vi "界面2-数据采集.vi"() -> ()   [LabVIEW 2013]
uses:
  GlobleVar/SamplingRate.vi
  GlobleVar/segment_size.vi
panel:
  out "CH2输出电流":dbl format="%.1f mA"
  in  "输出增益百分比-显示":dbl format="%.1f %"
  out "CH1输出电流":dbl format="%.1f mA"
  in  "DEH类型发送":bool
  in  "DEH内置参数发送":bool
  in  "DEH内置参数值":dbl caption="内置参数值" format="%.1f %"
  in  "DEH类型":enum32{"内置", "外接"}(radio) caption="类型"
  in  "无输出":bool
  in  "阀门全关":bool
  in  "阀门全开":bool
  in  "输出增益百分比":sgl(slide) scale=0.0..100.0
  out "total_size":dbl format="%#_6p"
  in  "采集结束":bool
  out "Boolean":bool
  in  "试验结果->":bool
  in  "<-项目":bool
  in  "中止":bool
  in  "开始":bool
  in  "完成":bool
  out "采集进度":u8 format="%0.0f%%"
  out "采集\n进度":u8(slide) scale=0.0..100.0
  in  "采样时间":dbl=4.0 format="%#_g s"
  in  "试验模式":u16(ring) items=["快关L1L2", "快关L1", "快关L2", "步响应1", "归零", "开启关闭"]
  out "实时采集":cluster{dbl, dbl, dbl[][]}(graph)
  # "DEH"
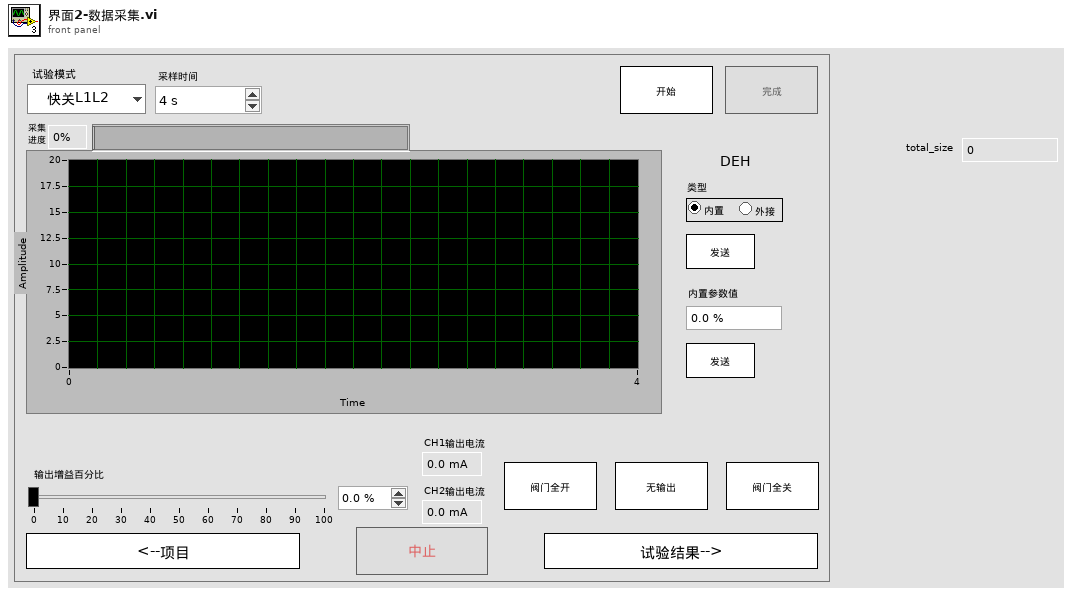
[diagram p1: front panel]
types:
  T1 = enum16{"初始化", "等待事件", "退出", "数据采集", "数据处理", "开启阀门"}
  T2 = cluster{"联机状态":bool, "外置清零信号":bool, "卡件工作模式":enum16{"无输出", "正常工作", "阀门常开", "阀门常闭"}, "卡件序列号":string, "卡件物理地址":string, "伺服阀输出电流CH1":dbl, "输出通道状态CH1":bool, "伺服阀输出电流CH2":dbl, "输出通道状态CH2":bool, "伺服输出使能CH1 ":bool, "伺服输出使能CH2":bool, "LVDT1类型":enum16{"未接入", "直流", "交流"}, "LVDT1直流回路":bool, "LVDT1次级线圈 2":bool, "LVDT1次级线圈 1":bool, "LVDT1初级线圈":bool, "LVDT2类型":enum16{"未接入", "直流", "交流"}, "LVDT2直流回路":bool, "LVDT2次级线圈 2":bool, "LVDT2次级线圈 1":bool, "LVDT2初级线圈":bool, "DEH回路状态":bool, "DEH类型":enum16{"内置", "外接"}, "转速反馈使能":bool, "LVDT1信号采样百分比":dbl, "LVDT2信号采样百分比":dbl, "DEH指令值":u8, "转速差反馈量":dbl, "回路1转速":dbl, "回路2转速":dbl, "回路3转速":dbl, "中选转速":dbl, "LVDT1 ADC":i16, "LVDT2 ADC":i16, "DEH ADC":i16, "LVDT1ZADC":i16, "LVDT2ZADC":i16, "LVDT1FADC":i16, "LVDT2FADC":i16, "DehZeroCali":bool, "DehFullCali":bool, "LVDT1ZeroCali":bool, "LVDT1FullCali":bool, "LVDT2ZeroCali":bool, "LVDT2FullCali":bool, "转速零度标定":i16, "转速满度标定":i16, "转速指令采样值":i16, "标准转速":dbl}
  T3 = enum8{"Enabled", "Disabled", "Disabled and Grayed Out"}
  T4 = enum16{"open", "open or create", "create or replace", "create", "open (read-only)"}
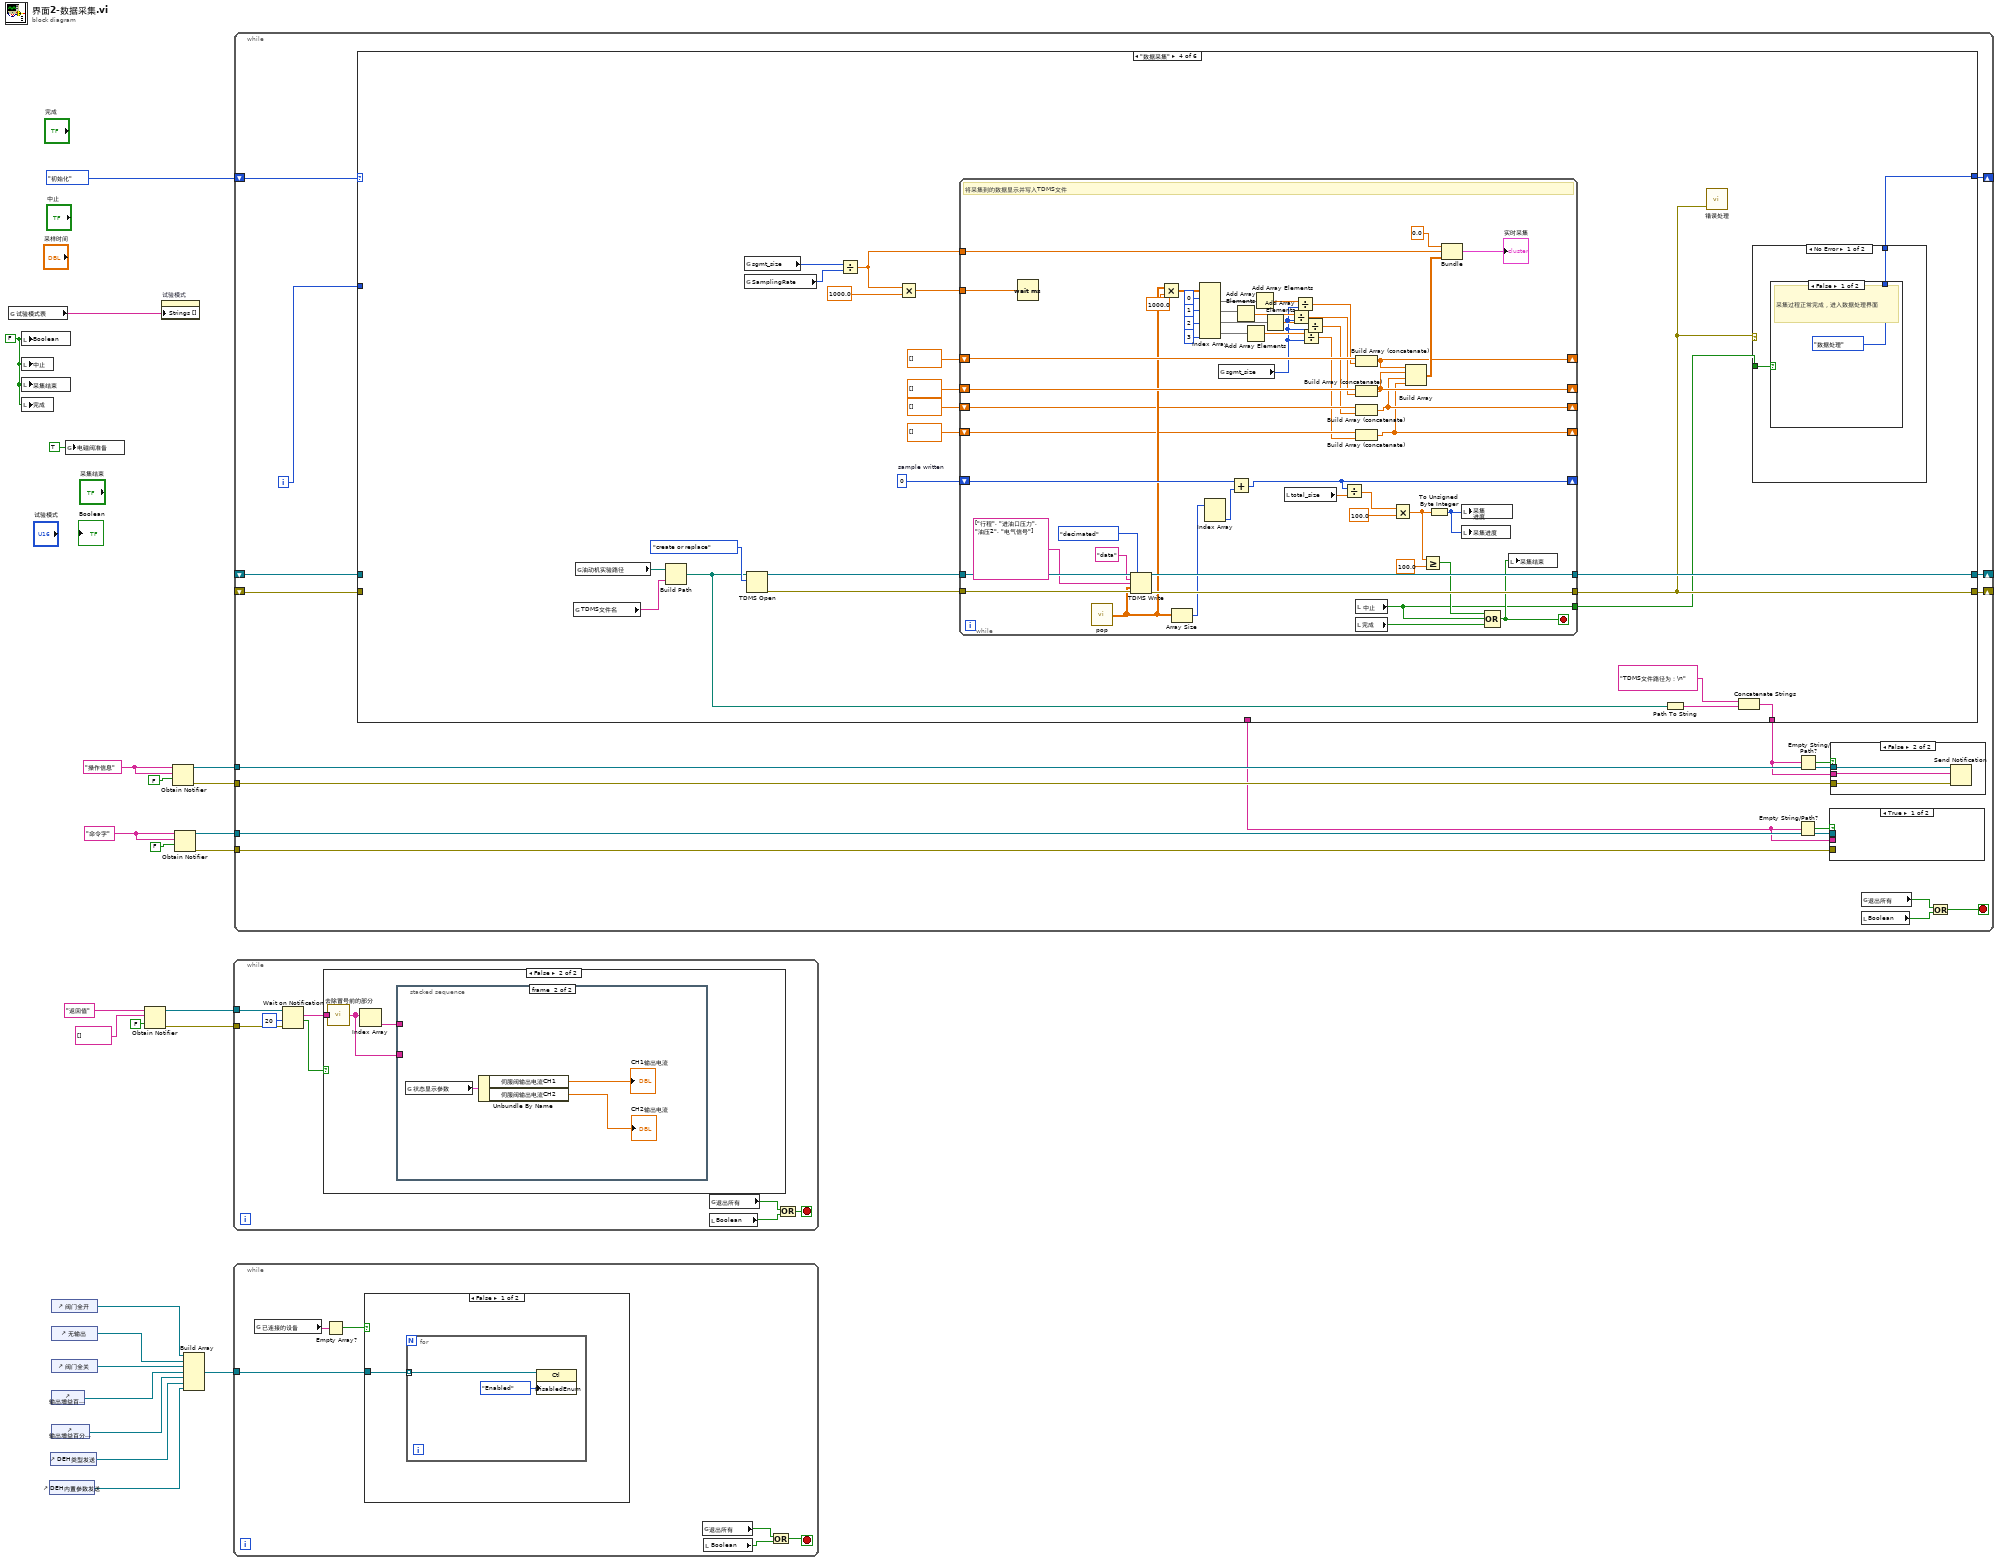
[diagram p0: block diagram]
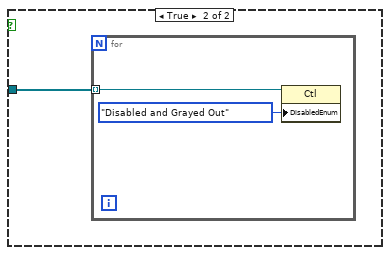
[diagram p2: hidden frame]
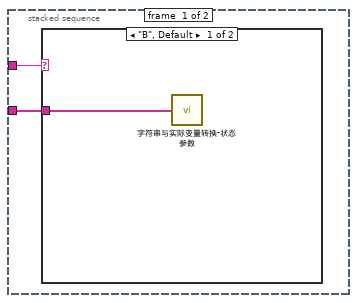
[diagram p4: hidden frame]
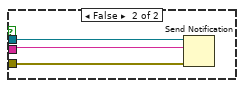
[diagram p6: hidden frame]
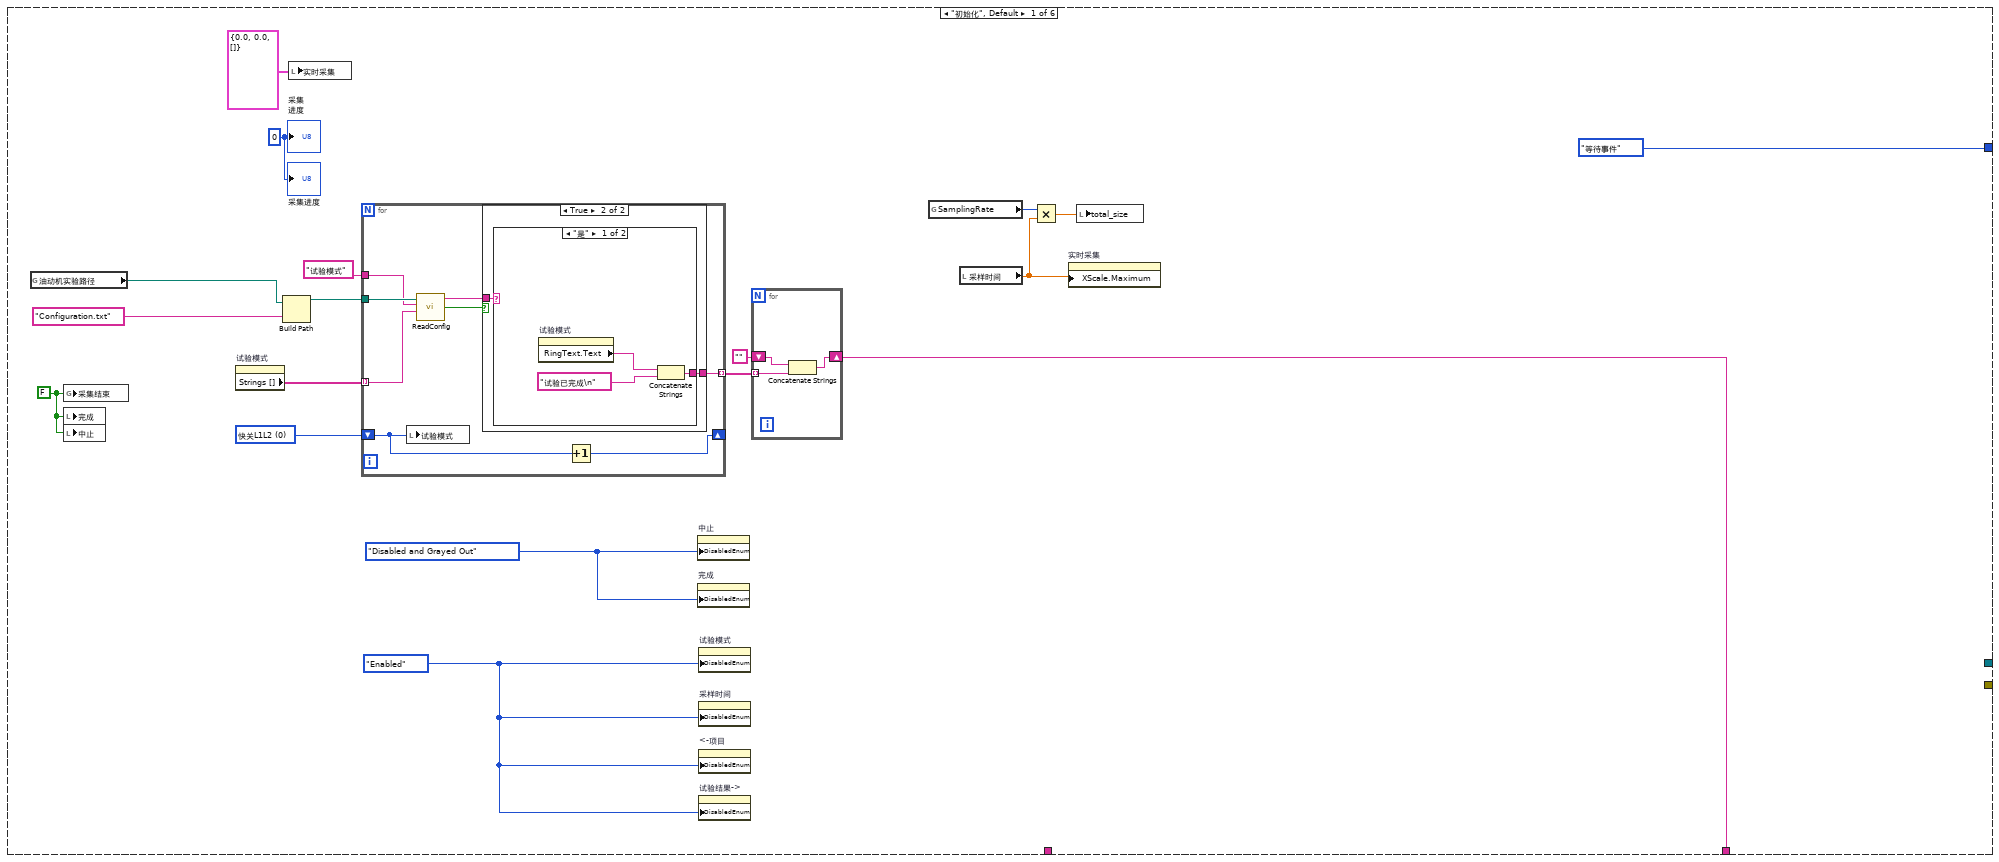
[diagram p8: hidden frame]
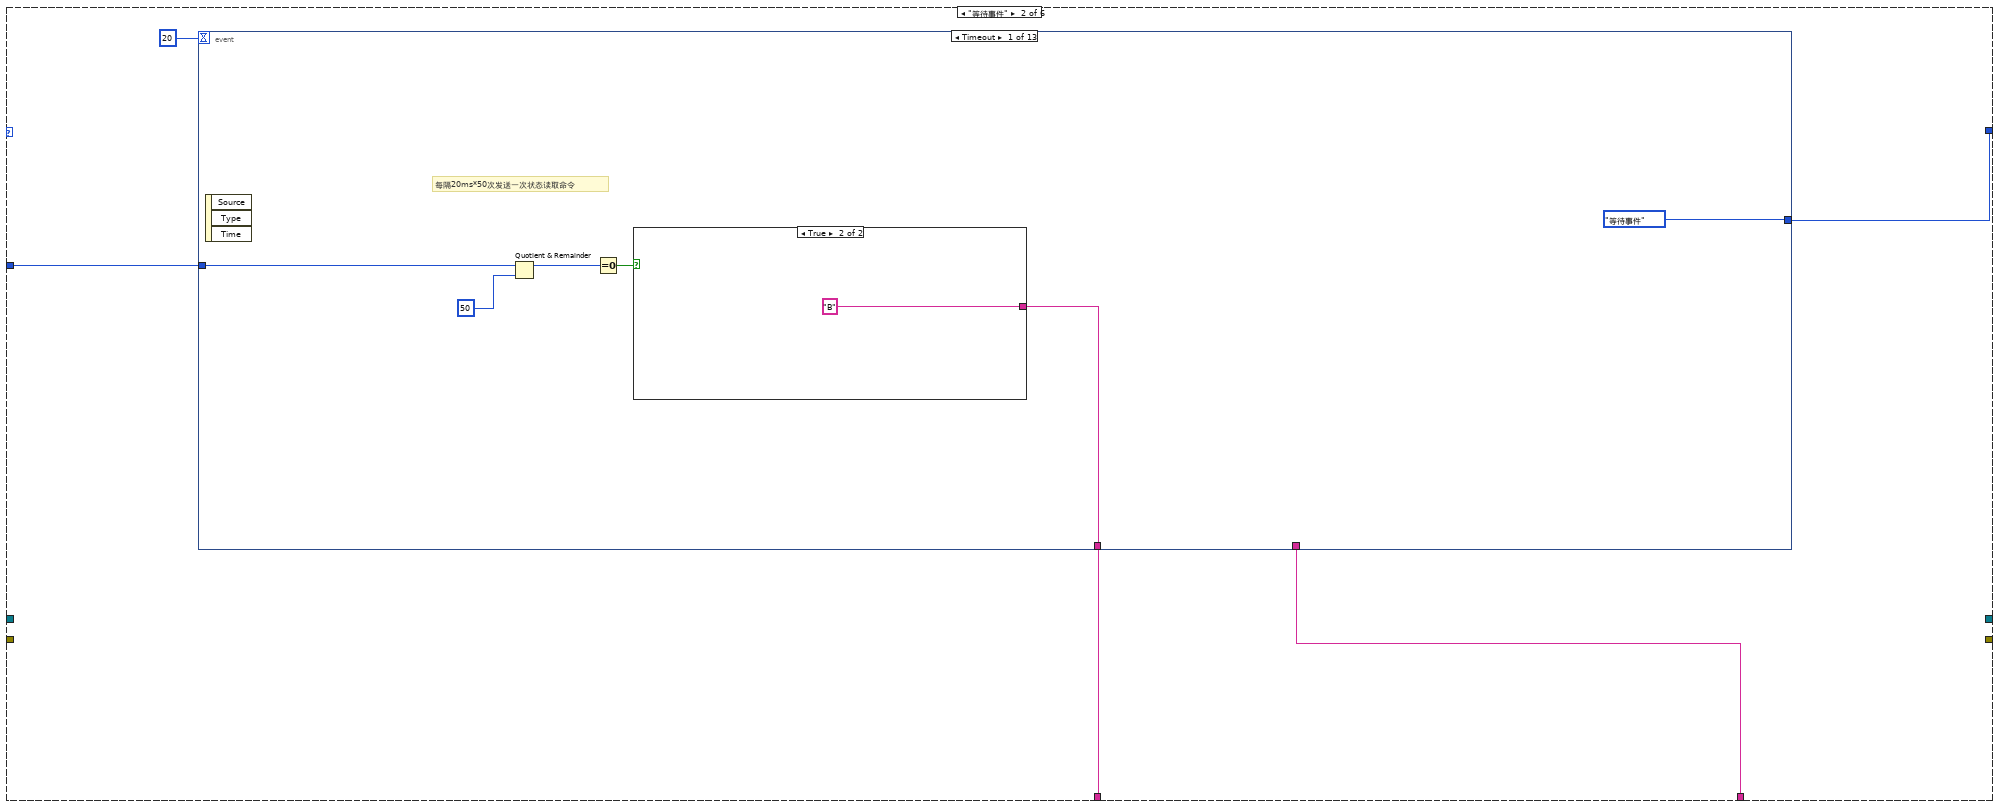
[diagram p11: hidden frame]
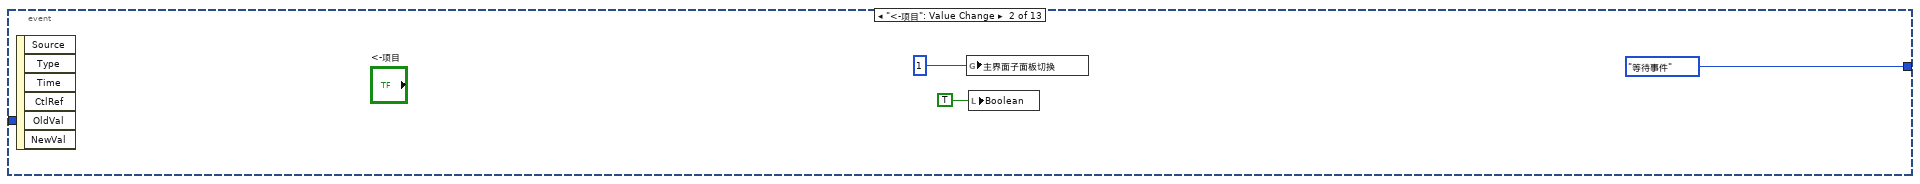
[diagram p13: hidden frame]
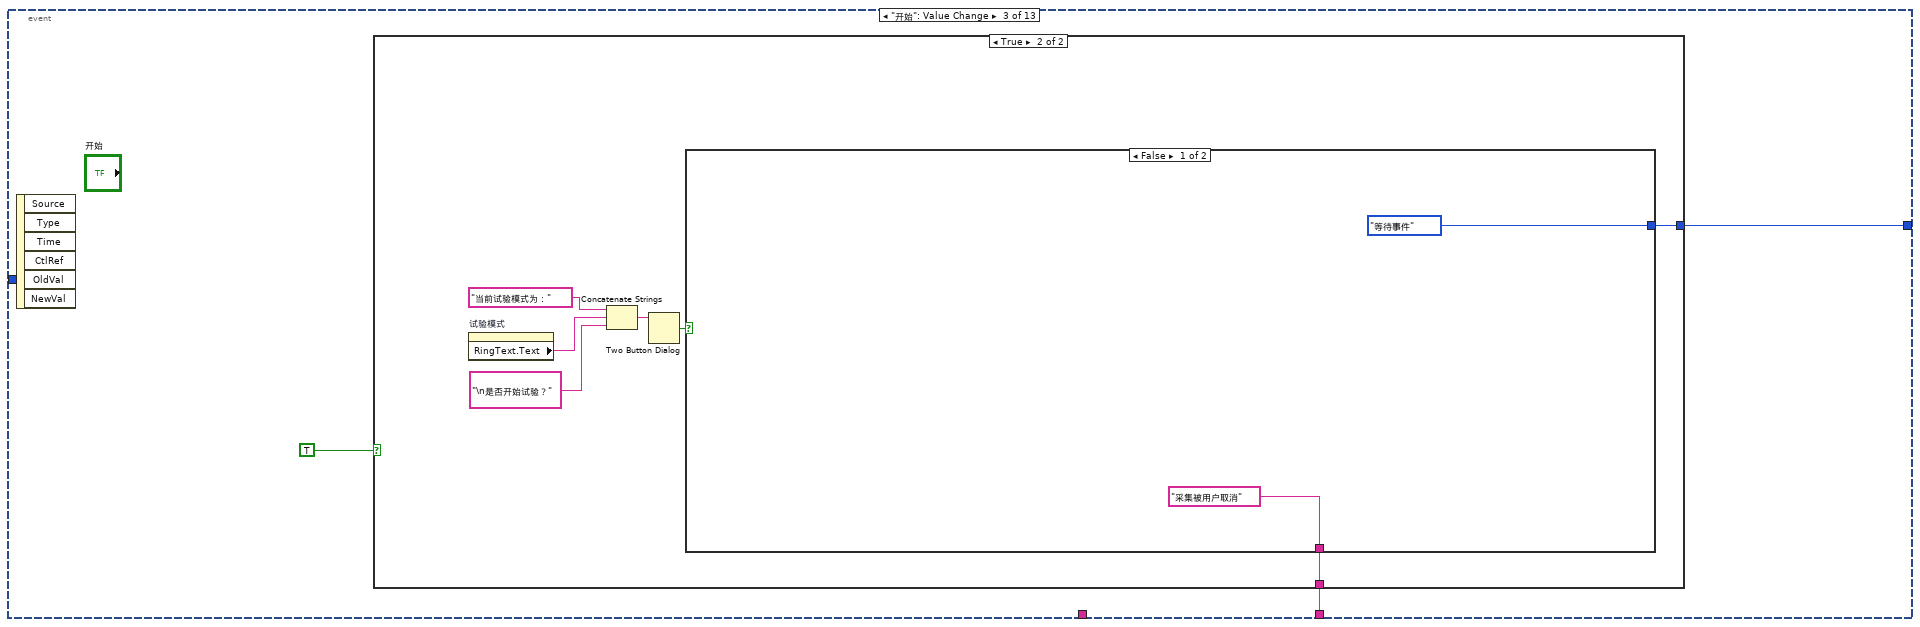
[diagram p14: hidden frame]
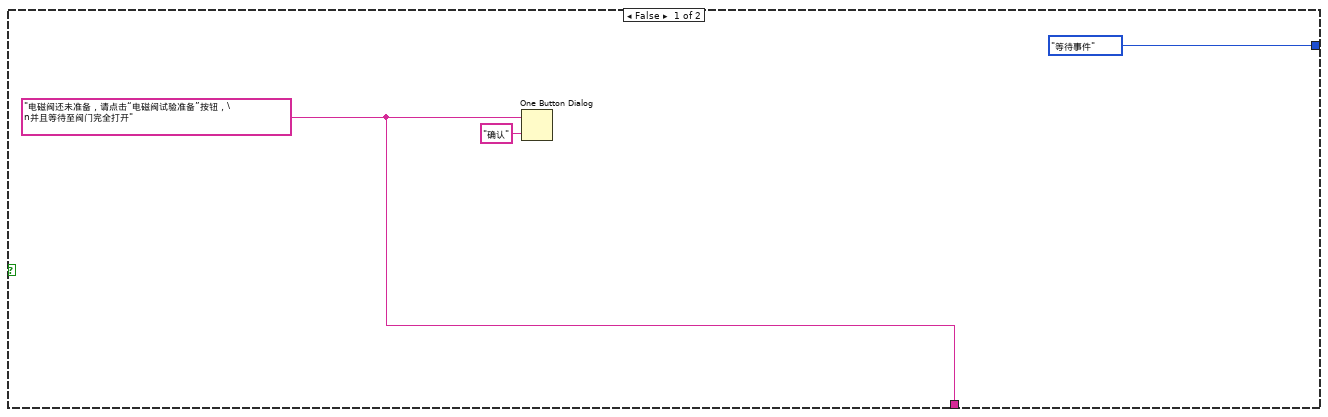
[diagram p15: hidden frame]
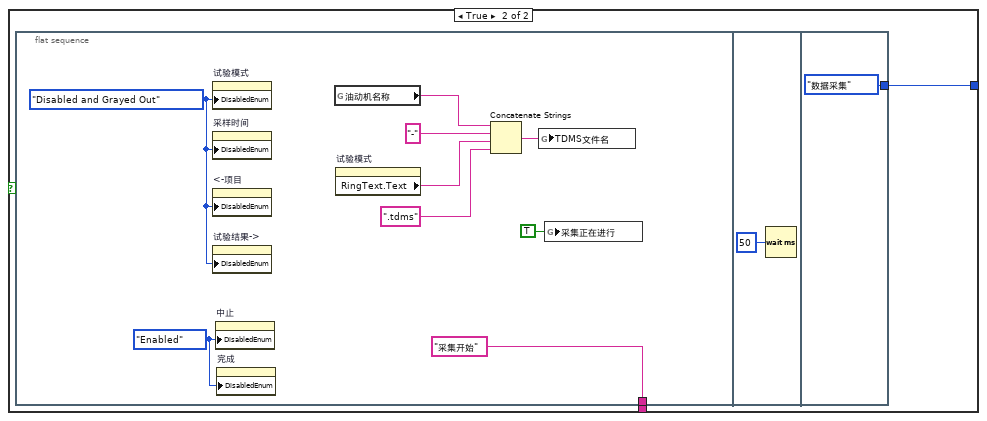
[diagram p16: hidden frame]
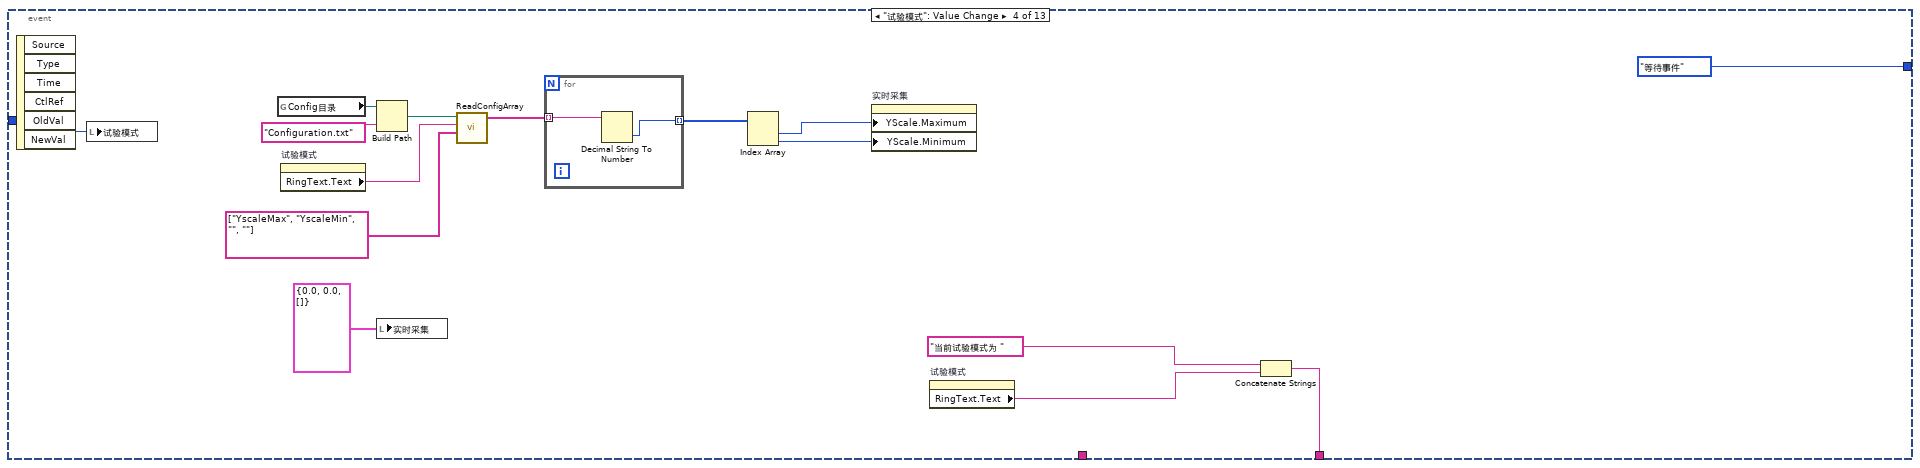
[diagram p17: hidden frame]
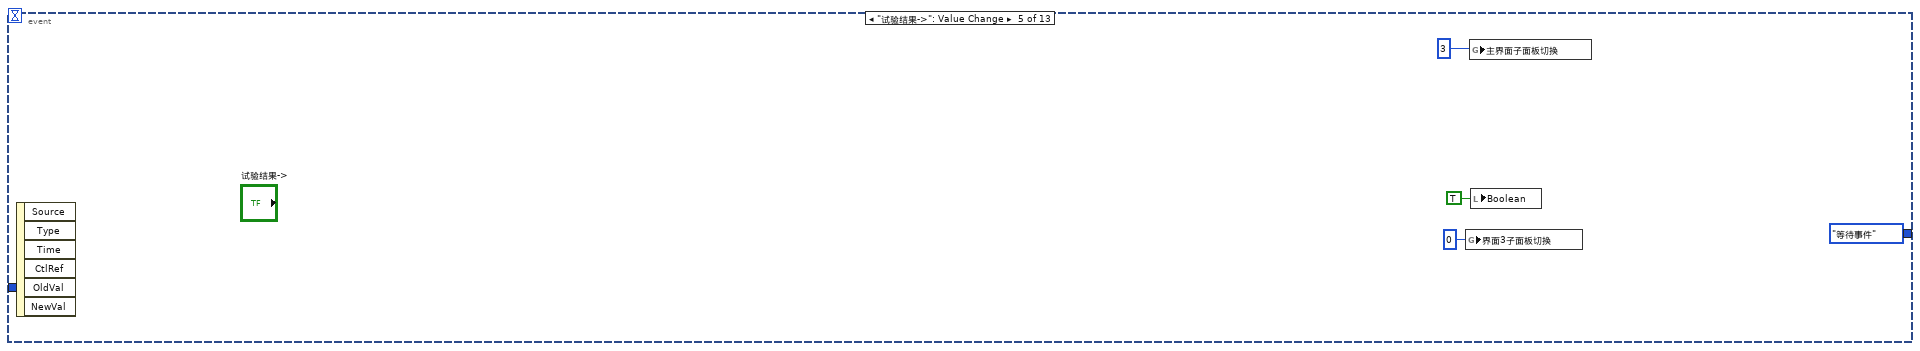
[diagram p18: hidden frame]
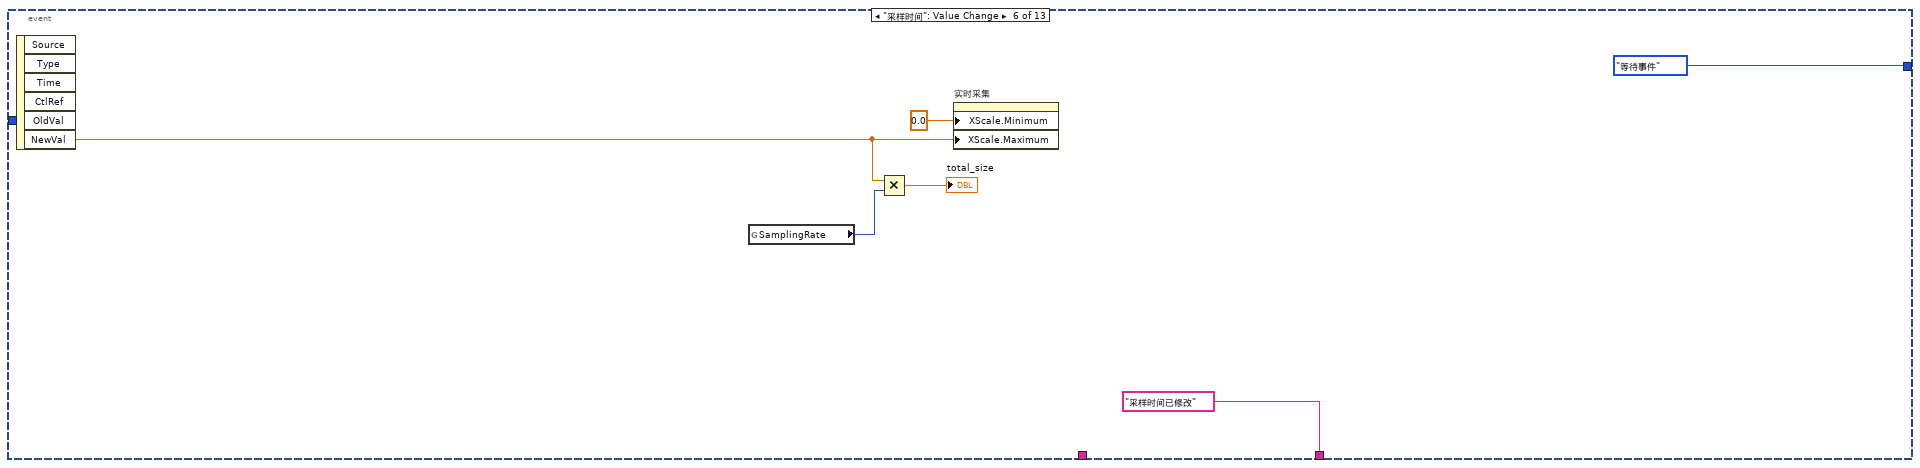
[diagram p19: hidden frame]
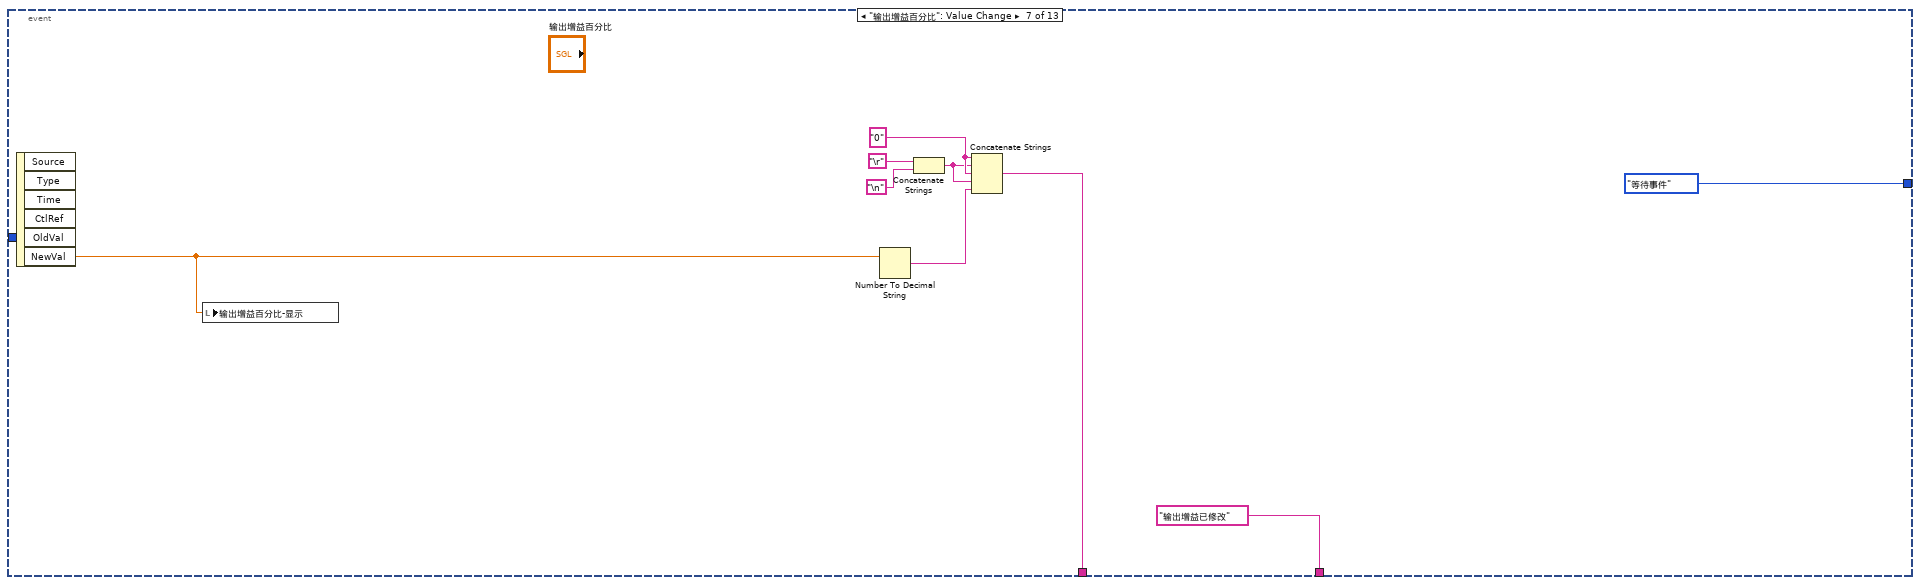
[diagram p20: hidden frame]
diagram:
  w16 = "命令字"
  w19 = FALSE ("Boolean")
  w24 = "操作信息"
  n1 = global read "试验模式表.vi" "试验模式表"() -> (w20:string[])
  n2 = local write "Boolean"(w19) -> ()
  n3 = local write "中止"(w19) -> ()
  n4 = local write "采集结束"(w19) -> ()
  n5 = local write "完成"(w19) -> ()
  n6 = control-ref of="DEH内置参数发送"() -> (w1:refnum<vi>)
  n7 = control-ref of="DEH类型发送"() -> (w2:refnum<vi>)
  n8 = control-ref of="阀门全开"() -> (w8:refnum<vi>)
  n9 = control-ref of="无输出"() -> (w7:refnum<vi>)
  n10 = control-ref of="阀门全关"() -> (w6:refnum<vi>)
  n11 = control-ref of="输出增益百分比"() -> (w5:refnum<vi>)
  n12 = control-ref of="输出增益百分比-显示"() -> (w4:refnum<vi>)
  n13 = global write "电磁阀准备.vi" "电磁阀准备"(TRUE ("电磁阀准备")) -> ()
  n14 = Obtain Notifier(name (unnamed)="返回值", notification data type=string[] [], create if not found? (T)=FALSE) -> (notifier out=w11:refnum<notifier>, error out=w10:errorcluster)  [unwired: 1 in, 1 out]
  n15 = property on="试验模式" class="Ring (strict)"("Strings []"=w20) -> ()  [unwired: 2 in, 2 out]
  n16 = Obtain Notifier(name (unnamed)=w24, notification data type=w24, create if not found? (T)=FALSE) -> (notifier out=w23:refnum<notifier>, error out=w22:errorcluster)  [unwired: 1 in, 1 out]
  n17 = Obtain Notifier(name (unnamed)=w16, notification data type=w16, create if not found? (T)=FALSE) -> (notifier out=w15:refnum<notifier>, error out=w14:errorcluster)  [unwired: 1 in, 1 out]
  n18 = Build Array(w8, w7, w6, w5, w4, w2, w1) -> (w3:refnum<vi>[])
  n19 = while {
    tunnel: w11 -> [w32]
    tunnel: w10 -> [w31]
    stop <- w28 stop-if-true
    n20 = Wait on Notification(notifier=w32, timeout in ms (-1)=20, error in (no error)=w31) -> (notification=w30:string[], timed out?=w26:bool)  [unwired: 1 in, 2 out]
    n21 = case shown="False" w26 {
      tunnel: w30 -> [_ w36]
      frame True {
      }
      frame False {
        n22 = call "去除冒号前的部分.vi"("返回值列表"=w36) -> ("返回值参数列表"=w34:string[])
        n23 = Index Array(array=w34) -> (element=w35:string)  [unwired: 1 in]
        n24 = stacked-sequence {
          tunnel: w35 -> [w38 _]
          tunnel: w34 -> [w37 _]
          frame #0 {
            n25 = case shown="\"B\", Default" w38 {
              tunnel: w37 -> [w39 _]
              frame "B", Default {
                n26 = call "字符串与实际变量转换-状态参数.vi"("状态参数"=w39) -> ()  [unwired: 5 in]
              }
              frame "True" {
              }
            }
          }
          frame #1 {
            n27 = global read "状态显示参数.vi" "状态显示参数"() -> (w42:T2)
            n28 = Unbundle By Name(w42) -> ("伺服阀输出电流CH1"=→"CH1输出电流":dbl, "伺服阀输出电流CH2"=→"CH2输出电流":dbl)
          }
        }
      }
    }
    n29 = global read "退出所有.vi" "退出所有"() -> (w29:bool)
    n30 = local read "Boolean"() -> (w27:bool)
    n31 = Or(x=w29, y=w27) -> (x .or. y?=w28:bool)
  }
  n32 = while {
    tunnel: w3 -> [w46]
    stop <- w44 stop-if-true
    n33 = global read "已连接的设备.vi" "已连接的设备"() -> (w48:string[])
    n34 = Empty Array?(array=w48) -> (empty?=w47:bool)
    n35 = case shown="False" w47 {
      tunnel: w46 -> [w49 w52]
      frame False {
        n36 = for {
          tunnel: w49 -> [w51] mode=indexing
          n37 = property class="Ctl"(reference=w51, "DisabledEnum"=T3."Enabled" ("Disabled")) -> ()  [unwired: 1 in, 2 out]
        }
      }
      frame True {
        n38 = for {
          tunnel: w52 -> [w54] mode=indexing
          n39 = property class="Ctl"(reference=w54, "DisabledEnum"=T3."Disabled and Grayed Out" ("Disabled")) -> ()  [unwired: 1 in, 2 out]
        }
      }
    }
    n40 = global read "退出所有.vi" "退出所有"() -> (w45:bool)
    n41 = local read "Boolean"() -> (w43:bool)
    n42 = Or(x=w45, y=w43) -> (x .or. y?=w44:bool)
  }
  n43 = while {
    shift-right: [w70] -> _
    shift-left: T1."初始化" -> [w71]
    tunnel: w23 -> [w72]
    tunnel: w22 -> [w60]
    shift-right: [w64] -> _
    shift-left: _ -> [w62]
    shift-right: [w63] -> _
    shift-left: _ -> [w61]
    tunnel: w15 -> [w58]
    tunnel: w14 -> [w56]
    i -> [w55]
    stop <- w67 stop-if-true
    n44 = case shown="\"数据采集\"" w71 {
      tunnel: [w86 w116 w253 w281 "数据处理完成" "阀门已开启"] -> w65
      tunnel: [enum16{"初始化", "等待事件", "退出"}."等待事件" w117 T1."初始化" w282 T1."等待事件" T1."数据采集"] -> w70
      tunnel: [_ _ _ w283 _ _] -> w64
      tunnel: [_ _ _ w280 _ _] -> w63
      tunnel: w62 -> [_ _ w255 _ w353 _]
      tunnel: w61 -> [_ _ w254 _ w352 _]
      tunnel: [_ w114 _ _ _ _] -> w57
      tunnel: w55 -> [_ w113 _ _ _ _]
      frame "初始化", Default {
        w82 = T3."Disabled and Grayed Out" ("Disabled")
        w83 = T3."Enabled" ("Disabled")
        w89 = u16 0 items=["快关L1L2", "快关L1", "快关L2", "步响应", "归零", "开启关闭", ""] ("试验模式")
        w85 = FALSE
        w95 = u8 0 ("采集\n进度")
        n45 = global read "油动机实验路径.vi" "油动机实验路径"() -> (w93:path)
        n46 = global write "采集结束.vi" "采集结束"(w85) -> ()
        n47 = local write "完成"(w85) -> ()
        n48 = local write "中止"(w85) -> ()
        n49 = property on="试验模式" class="Ring (strict)"() -> ("Strings []"=w90:string[])  [unwired: 2 in, 2 out]
        n50 = Build Path(base path=w93, name or relative path="Configuration.txt" ("名称或相对路径")) -> (appended path=w92:path)
        n51 = local write "实时采集"(cluster{dbl, dbl, dbl[][]} {0.0, 0.0, []} ("实时采集")) -> ()
        n52 = for {
          tunnel: w92 -> [w107]
          tunnel: "试验模式" -> [w106]
          tunnel: w90 -> [w105] mode=indexing
          shift-right: [w101] -> _
          shift-left: w89 -> [w102]
          tunnel: [w100] -> w87 mode=indexing
          n53 = local write "试验模式"(w102) -> ()
          n54 = call "ReadConfig.vi"("Key"=w105, "Section"=w106, "Path"=w107) -> ("Key found?"=w104:bool, "Value"=w103:string)  [unwired: 1 in, 1 out]
          n55 = case shown="True" w104 {
            tunnel: w103 -> [_ w109]
            tunnel: [_ w108] -> w100
            frame False {
            }
            frame True {
              n56 = case shown="\"是\"" w109 {
                tunnel: [w110 _] -> w108
                frame "是" {
                  n57 = property on="试验模式" class="Ring (strict)"() -> ("RingText.Text"=w111:string)  [unwired: 2 in, 2 out]
                  n58 = Concatenate Strings(w111, "试验已完成\n") -> (w110:string)
                }
                frame "否", Default {
                }
              }
            }
          }
          n59 = Increment(x=w102) -> (x+1=w101:u16)
        }
        n60 = property on="中止" class="Bool (strict)"("DisabledEnum"=w82) -> ()  [unwired: 2 in, 2 out]
        n61 = property on="完成" class="Bool (strict)"("DisabledEnum"=w82) -> ()  [unwired: 2 in, 2 out]
        n62 = property on="试验模式" class="Ring (strict)"("DisabledEnum"=w83) -> ()  [unwired: 2 in, 2 out]
        n63 = property on="采样时间" class="DigNum (strict)"("DisabledEnum"=w83) -> ()  [unwired: 2 in, 2 out]
        n64 = property on="<-项目" class="Bool"("DisabledEnum"=w83) -> ()  [unwired: 2 in, 2 out]
        n65 = property on="试验结果->" class="Bool"("DisabledEnum"=w83) -> ()  [unwired: 2 in, 2 out]
        n66 = for {
          shift-right: [w97] -> w86
          shift-left: "" -> [w98]
          tunnel: w87 -> [w99] mode=indexing
          n67 = Concatenate Strings(w98, w99) -> (w97:string)
        }
        n68 = global read "SamplingRate.vi" "SamplingRate"() -> (w79:i32)
        n69 = local read "采样时间"() -> (w80:dbl)
        n70 = Multiply(x=w79, y=w80) -> (x*y=w81:dbl)
        n71 = property on="实时采集" class="WFGraph (strict)"("XScale.Maximum"=w80) -> ()  [unwired: 2 in, 2 out]
        n72 = local write "total_size"(w81) -> ()
        "采集\n进度" <- w95
        "采集进度" <- w95
      }
      frame "等待事件" {
        n73 = event shown="[0] Timeout" {
          selector: _ -> [_ _ _ _ _ _ _ _ _ _ _ _ _]
          dyn-events: _ -> [_ _ _ _ _ _ _ _ _ _ _ _ _]
          timeout: 20 -> [_ _ _ _ _ _ _ _ _ _ _ _ _]
          tunnel: [T1."等待事件" T1."等待事件" w130 T1."等待事件" T1."等待事件" T1."等待事件" T1."等待事件" T1."等待事件" T1."等待事件" T1."等待事件" T1."等待事件" T1."等待事件" T1."等待事件"] -> w117
          tunnel: [_ _ w129 w167 _ "采样时间已修改" "输出增益已修改" ("消息") "输出增益已修改" ("消息") "无输出命令已发送" ("消息") "阀门全开命令已发送" ("消息") "阀门全关命令已发送" ("消息") w229 "DEH内置参数已发送" ("消息")] -> w116
          tunnel: [w118 _ _ _ _ _ w186 w195 w203 w218 w221 w234 w246] -> w114
          tunnel: w113 -> [w122 _ _ _ _ _ _ _ _ _ _ _ _]
          event Timeout {
            # "每隔20ms*50次发送一次状态读取命令"
            n74 = event-data() -> ()  [unwired: 1 in, 3 out]
            n75 = Quotient & Remainder(x=w122, y=50) -> (x-y*floor(x/y)=w119:i32)  [unwired: 1 out]
            n76 = Equal To 0?(x=w119) -> (x = 0?=w120:bool)
            n77 = case shown="True" w120 {
              tunnel: [_ "B"] -> w118
              frame False {
              }
              frame True {
              }
            }
          }
          event "<-项目": Value Change {
            n78 = event-data() -> ()  [unwired: 1 in, 6 out]
            n79 = global write "主界面子面板切换.vi" "主界面子面板切换"(1) -> ()
            n80 = local write "Boolean"(TRUE ("Boolean")) -> ()
          }
          event "开始": Value Change {
            n81 = event-data() -> ()  [unwired: 1 in, 6 out]
            n82 = case shown="True" TRUE {
              tunnel: [T1."等待事件" w140] -> w130
              tunnel: [w131 w134] -> w129
              frame False {
                w131 = "电磁阀还未准备，请点击“电磁阀试验准备”按钮，\n并且等待至阀门完全打开" ("消息")
                n83 = One Button Dialog(message=w131, button name ("OK")="确认") -> ()  [unwired: 1 out]
              }
              frame True {
                n84 = property on="试验模式" class="Ring (strict)"() -> ("RingText.Text"=w138:string)  [unwired: 2 in, 2 out]
                n85 = Concatenate Strings("当前试验模式为：", w138, "\n是否开始试验？") -> (w136:string)
                n86 = Two Button Dialog(message=w136) -> (T button?=w135:bool)  [unwired: 2 in]
                n87 = case shown="False" w135 {
                  tunnel: [T1."等待事件" w143] -> w140
                  tunnel: ["采集被用户取消" w144] -> w134
                  frame False {
                  }
                  frame True {
                    n88 = flat-sequence {
                      tunnel: ["采集开始"] -> w144
                      tunnel: [T1."数据采集"] -> w143
                      frame #0 {
                        w146 = T3."Enabled" ("Disabled")
                        w147 = T3."Disabled and Grayed Out" ("Disabled")
                        n89 = property on="试验模式" class="Ring (strict)"("DisabledEnum"=w147) -> ()  [unwired: 2 in, 2 out]
                        n90 = property on="采样时间" class="DigNum (strict)"("DisabledEnum"=w147) -> ()  [unwired: 2 in, 2 out]
                        n91 = property on="<-项目" class="Bool"("DisabledEnum"=w147) -> ()  [unwired: 2 in, 2 out]
                        n92 = property on="试验结果->" class="Bool"("DisabledEnum"=w147) -> ()  [unwired: 2 in, 2 out]
                        n93 = property on="中止" class="Bool (strict)"("DisabledEnum"=w146) -> ()  [unwired: 2 in, 2 out]
                        n94 = property on="完成" class="Bool (strict)"("DisabledEnum"=w146) -> ()  [unwired: 2 in, 2 out]
                        n95 = global read "油动机名称.vi" "油动机名称"() -> (w149:string)
                        n96 = property on="试验模式" class="Ring (strict)"() -> ("RingText.Text"=w151:string)  [unwired: 2 in, 2 out]
                        n97 = Concatenate Strings(w149, "-", w151, ".tdms") -> (w153:string)
                        n98 = global write "TDMS文件名.vi" "TDMS文件名"(w153) -> ()
                        n99 = global write "采集正在进行.vi" "采集正在进行"(TRUE ("采集正在进行")) -> ()
                      }
                      frame #1 {
                        n100 = Wait (ms)(milliseconds to wait=u32 50) -> ()  [unwired: 1 out]
                      }
                      frame #2 {
                      }
                    }
                  }
                }
              }
            }
          }
          event "试验模式": Value Change {
            n101 = event-data() -> ("NewVal"=w170:u16)  [unwired: 1 in, 5 out]
            n102 = local write "试验模式"(w170) -> ()
            n103 = global read "Config目录.vi" "Config目录"() -> (w164:path)
            n104 = property on="试验模式" class="Ring (strict)"() -> ("RingText.Text"=w162:string)  [unwired: 2 in, 2 out]
            n105 = Build Path(base path=w164, name or relative path="Configuration.txt") -> (appended path=w165:path)
            n106 = local write "实时采集"(cluster{dbl, dbl, dbl[][]} {0.0, 0.0, []} ("实时采集")) -> ()
            n107 = call "ReadConfigArray.vi"("KeyArray"=string[] ["YscaleMax", "YscaleMin", "", ""], "Section"=w162, "Path"=w165) -> ("ValueArray"=w160:string[])  [unwired: 1 in, 2 out]
            n108 = for {
              tunnel: w160 -> [w172] mode=indexing
              tunnel: [w171] -> w159 mode=indexing
              n109 = Decimal String To Number(string=w172) -> (number=w171:i32)  [unwired: 2 in, 1 out]
            }
            n110 = Index Array(array=w159) -> (element #1=w158:i32, element #2=w157:i32)  [unwired: 2 in]
            n111 = property on="实时采集" class="WFGraph (strict)"("YScale.Maximum"=w158, "YScale.Minimum"=w157) -> ()  [unwired: 2 in, 2 out]
            n112 = property on="试验模式" class="Ring (strict)"() -> ("RingText.Text"=w168:string)  [unwired: 2 in, 2 out]
            n113 = Concatenate Strings("当前试验模式为 ", w168) -> (w167:string)
          }
          event "试验结果->": Value Change {
            n114 = event-data() -> ()  [unwired: 1 in, 6 out]
            n115 = global write "界面3子面板切换.vi" "界面3子面板切换"(0 ("界面3子面板切换")) -> ()
            n116 = global write "主界面子面板切换.vi" "主界面子面板切换"(3) -> ()
            n117 = local write "Boolean"(TRUE ("Boolean")) -> ()
          }
          event "采样时间": Value Change {
            n118 = event-data() -> ("NewVal"=w181:dbl)  [unwired: 1 in, 5 out]
            n119 = global read "SamplingRate.vi" "SamplingRate"() -> (w178:i32)
            n120 = Multiply(x=w181, y=w178) -> (x*y=→"total_size":dbl)
            n121 = property on="实时采集" class="WFGraph (strict)"("XScale.Minimum"=0.0 ("X Scale.Range:Minimum"), "XScale.Maximum"=w181) -> ()  [unwired: 2 in, 2 out]
          }
          event "输出增益百分比": Value Change {
            w189 = "0"
            n122 = event-data() -> ("NewVal"=w183:sgl)  [unwired: 1 in, 5 out]
            n123 = local write "输出增益百分比-显示"(w183) -> ()
            n124 = Number To Decimal String(number=w183) -> (decimal integer string=w187:string)  [unwired: 1 in]
            n125 = Concatenate Strings("\r", "\n") -> (w188:string)
            n126 = Concatenate Strings(w189, w188, w189, w188, w187) -> (w186:string)
          }
          event "输出增益百分比-显示": Value Change {
            w198 = "0"
            n127 = event-data() -> ("NewVal"=w194:dbl)  [unwired: 1 in, 5 out]
            n128 = local write "输出增益百分比"(w194) -> ()
            n129 = Number To Decimal String(number=w194) -> (decimal integer string=w196:string)  [unwired: 1 in]
            n130 = Concatenate Strings("\r", "\n") -> (w197:string)
            n131 = Concatenate Strings(w198, w197, w198, w197, w196) -> (w195:string)
          }
          event "无输出": Value Change {
            n132 = event-data() -> ()  [unwired: 1 in, 6 out]
            n133 = Concatenate Strings("\r", "\n") -> (w206:string)
            n134 = Concatenate Strings("0", w206, "1", w206, "0") -> (w203:string)
          }
          event "阀门全开": Value Change {
            n135 = event-data() -> ()  [unwired: 1 in, 6 out]
            n136 = Concatenate Strings("\r", "\n") -> (w214:string)
            n137 = Concatenate Strings("0", w214, "1", w214, "2") -> (w218:string)
          }
          event "阀门全关": Value Change {
            n138 = event-data() -> ()  [unwired: 1 in, 6 out]
            n139 = Concatenate Strings("\r", "\n") -> (w224:string)
            n140 = Concatenate Strings("0", w224, "1", w224, "3") -> (w221:string)
          }
          event "DEH类型发送": Value Change {
            n141 = event-data() -> ()  [unwired: 1 in, 6 out]
            n142 = Number To Decimal String(number="DEH类型") -> (decimal integer string=w233:string)  [unwired: 1 in]
            n143 = Concatenate Strings("\r", "\n") -> (w236:string)
            n144 = Concatenate Strings("0", w236, "2", w236, w233) -> (w234:string)
            n145 = case shown="\"外接\"" "DEH类型" {
              tunnel: ["内置" "外接"] -> w230
              frame "内置", Default {
              }
              frame "外接" {
              }
            }
            n146 = Concatenate Strings("DEH设置为：" ("消息"), w230) -> (w229:string)
          }
          event "DEH内置参数发送": Value Change {
            n147 = event-data() -> ()  [unwired: 1 in, 6 out]
            n148 = Number To Fractional String(number="DEH内置参数值") -> (F-format string=w244:string)  [unwired: 3 in]
            n149 = Concatenate Strings("\r", "\n") -> (w247:string)
            n150 = Concatenate Strings("5", w247, w244) -> (w246:string)
          }
        }
      }
      frame "退出" {
        w251 = T3."Disabled and Grayed Out" ("Disabled")
        w252 = T3."Enabled" ("Disabled")
        n151 = flat-sequence {
          tunnel: w255 -> [w259]
          tunnel: w254 -> [w258]
          tunnel: ["TDMS和TDMS_index已删除"] -> w253
          frame #0 {
            n152 = TDMS Close(8:w258, 11:w259) -> ()  [unwired: 2 out]
            n153 = Wait (ms)(milliseconds to wait=u32 20) -> ()  [unwired: 1 out]
          }
          frame #1 {
            n154 = global read "油动机实验路径.vi" "油动机实验路径"() -> (w261:path)
            n155 = global read "TDMS文件名.vi" "TDMS文件名"() -> (w268:string)
            n156 = Build Path(base path=w261, name or relative path=w268) -> (appended path=w263:path)
            n157 = Path To String(path=w263) -> (string=w262:string)
            n158 = Concatenate Strings(w262, "_index" ("字符串")) -> (w266:string)
            n159 = String To Path(string=w262) -> (path=w264:path)
            n160 = String To Path(string=w266) -> (path=w265:path)
            n161 = Delete(path (use dialog)=w264) -> ()  [unwired: 4 in, 3 out]
            n162 = Delete(path (use dialog)=w265) -> ()  [unwired: 4 in, 3 out]
          }
        }
        n163 = property on="<-项目" class="Bool"("DisabledEnum"=w252) -> ()  [unwired: 2 in, 2 out]
        n164 = property on="采样时间" class="DigNum (strict)"("DisabledEnum"=w252) -> ()  [unwired: 2 in, 2 out]
        n165 = property on="试验模式" class="Ring (strict)"("DisabledEnum"=w252) -> ()  [unwired: 2 in, 2 out]
        n166 = property on="试验结果->" class="Bool"("DisabledEnum"=w252) -> ()  [unwired: 2 in, 2 out]
        n167 = property on="中止" class="Bool (strict)"("DisabledEnum"=w251) -> ()  [unwired: 2 in, 2 out]
        n168 = property on="完成" class="Bool (strict)"("DisabledEnum"=w251) -> ()  [unwired: 2 in, 2 out]
      }
      frame "数据采集" {
        w279 = 0  # sample written
        n169 = global read "TDMS文件名.vi" "TDMS文件名"() -> (w288:string)
        n170 = global read "油动机实验路径.vi" "油动机实验路径"() -> (w289:path)
        n171 = Build Path(base path=w289, name or relative path=w288) -> (appended path=w286:path)
        n172 = global read "segment_size.vi" "sgmt_size"() -> (w277:i32)
        n173 = global read "SamplingRate.vi" "SamplingRate"() -> (w276:i32)
        n174 = TDMS Open(10:T4."create or replace" ("operation (0:open)"), 11:w286) -> (0:w290:errorcluster, 3:w291:refnum<k34>)  [unwired: 5 in]
        n175 = Divide(x=w277, y=w276) -> (x/y=w271:dbl)
        n176 = Multiply(x=w271, y=1000.0) -> (x*y=w274:dbl)
        n177 = while {
          tunnel: w291 -> [w350]
          tunnel: w290 -> [w347]
          tunnel: [w349] -> w283
          tunnel: [w346] -> w280
          shift-right: [w335] -> _
          shift-left: w279 -> [w342]
          tunnel: [w331] -> w278
          tunnel: w274 -> [w323]
          shift-right: [w325] -> _
          shift-left: dbl[] [] -> [w327]
          shift-right: [w324] -> _
          shift-left: dbl[] [] -> [w326]
          tunnel: w271 -> [w322]
          shift-right: [w299] -> _
          shift-left: dbl[] [] -> [w302]
          shift-right: [w298] -> _
          shift-left: dbl[] [] -> [w303]
          stop <- w332 stop-if-true
          # "将采集到的数据显示并写入TDMS文件"
          n178 = Wait (ms)(milliseconds to wait=w323) -> ()  [unwired: 1 out]
          n179 = call "pop.vi"() -> ("Data out"=w319:dbl[][])  [unwired: 1 in]
          n180 = TDMS Write(0:w350, 1:enum16{"decimated", "interleaved"}."decimated" ("数据布局（0:降采样）"), 5:"data" ("组名称输入（无标题）"), 7:string[] ["行程", "进油口压力", "油压2", "电气信号"] ("通道名输入（无标题）"), 9:w319, 11:w347) -> (4:w349:refnum<k34>, 15:w346:errorcluster)  [unwired: 2 out]
          n181 = Multiply(x=w319, y=1000.0) -> (x*y=w318:dbl[][])
          n182 = Array Size(array=w319) -> (size(s)=w344:i32[])
          n183 = Index Array(array=w318, index (row) #1=0 ("disabled index (col)"), index (row) #2=1 ("index (row)"), index (row) #3=2 ("index (row)"), index (row) #4=3 ("index (row)")) -> (element #1=w321:dbl[], element #2=w320:dbl[], element #3=w306:dbl[], element #4=w305:dbl[])  [unwired: 4 in]
          n184 = Index Array(array=w344) -> (element #2=w343:i32)  [unwired: 2 in, 1 out]
          n185 = global read "segment_size.vi" "sgmt_size"() -> (w304:i32)
          n186 = Add(x=w342, y=w343) -> (x+y=w335:i32)
          n187 = Add Array Elements(numeric array=w320) -> (sum=w314:dbl)
          n188 = Add Array Elements(numeric array=w305) -> (sum=w307:dbl)
          n189 = Add Array Elements(numeric array=w321) -> (sum=w316:dbl)
          n190 = Add Array Elements(numeric array=w306) -> (sum=w308:dbl)
          n191 = local read "total_size"() -> (w336:dbl)
          n192 = Divide(x=w314, y=w304) -> (x/y=w313:dbl)
          n193 = Divide(x=w316, y=w304) -> (x/y=w315:dbl)
          n194 = Divide(x=w307, y=w304) -> (x/y=w300:dbl)
          n195 = Divide(x=w308, y=w304) -> (x/y=w301:dbl)
          n196 = Divide(x=w335, y=w336) -> (x/y=w339:dbl)
          n197 = local read "完成"() -> (w334:bool)
          n198 = Build Array (concatenate)(w327, w315) -> (w325:dbl[])
          n199 = Build Array (concatenate)(w326, w313) -> (w324:dbl[])
          n200 = Build Array (concatenate)(w302, w301) -> (w299:dbl[])
          n201 = Build Array (concatenate)(w303, w300) -> (w298:dbl[])
          n202 = local read "中止"() -> (w331:bool)
          n203 = Multiply(x=w339, y=100.0) -> (x*y=w340:dbl)
          n204 = Build Array(w325, w324, w299, w298) -> (w328:dbl[][])
          n205 = Greater Or Equal?(x=w340, y=100.0) -> (x >= y?=w333:bool)
          n206 = To Unsigned Byte Integer(number=w340) -> (unsigned 8bit integer=w337:u8)
          n207 = Bundle(0.0, w322, w328) -> (→"实时采集":cluster{dbl, dbl, dbl[][]})  [unwired: 1 in]
          n208 = local write "采集\n进度"(w337) -> ()
          n209 = local write "采集进度"(w337) -> ()
          n210 = Compound Arithmetic op=OR(w333, w331, w334) -> (w332:bool)
          n211 = local write "采集结束"(w332) -> ()
        }
        n212 = Path To String(path=w286) -> (string=w284:string)
        n213 = call "错误处理.vi"("error in (no error)"=w280) -> ()  [unwired: 2 in]
        n214 = Concatenate Strings("TDMS文件路径为：\n", w284) -> (w281:string)
        n215 = case shown="No Error" w280 {
          tunnel: w278 -> [w293 _]
          tunnel: [w292 T1."退出"] -> w282
          frame No Error {
            n216 = case shown="False" w293 {
              tunnel: [T1."数据处理" T1."退出"] -> w292
              frame False {
                # "采集过程正常完成，进入数据处理界面"
              }
              frame True {
                # "采集过程被用户中止，进入退出状态"
              }
            }
          }
          frame Error {
            n217 = Two Button Dialog(message="TDMS文件操作错误，请重新开始") -> ()  [unwired: 2 in, 1 out]
          }
        }
      }
      frame "数据处理" {
        w354 = T3."Disabled and Grayed Out" ("Disabled")
        w355 = T3."Enabled" ("Disabled")
        # "试验数据采集成功后进入数据处理阶段\n才更改configuration中的否为是"
        n218 = global read "油动机实验路径.vi" "油动机实验路径"() -> (w360:path)
        n219 = Build Path(base path=w360, name or relative path="Configuration.txt" ("名称或相对路径")) -> (appended path=w359:path)
        n220 = property on="试验模式" class="Ring (strict)"() -> ("RingText.Text"=w357:string)  [unwired: 2 in, 2 out]
        n221 = property on="试验模式" class="Ring (strict)"("DisabledEnum"=w355) -> ()  [unwired: 2 in, 2 out]
        n222 = property on="试验结果->" class="Bool"("DisabledEnum"=w355) -> ()  [unwired: 2 in, 2 out]
        n223 = property on="<-项目" class="Bool"("DisabledEnum"=w355) -> ()  [unwired: 2 in, 2 out]
        n224 = property on="采样时间" class="DigNum (strict)"("DisabledEnum"=w355) -> ()  [unwired: 2 in, 2 out]
        n225 = property on="中止" class="Bool (strict)"("DisabledEnum"=w354) -> ()  [unwired: 2 in, 2 out]
        n226 = property on="完成" class="Bool (strict)"("DisabledEnum"=w354) -> ()  [unwired: 2 in, 2 out]
        n227 = call "Write2Config.vi"("Path"=w359, "Section"="试验模式" ("section"), "Key"=w357, "Value"="是") -> ()  [unwired: 11 in, 1 out]
        n228 = TDMS Close(8:w352, 11:w353) -> ()  [unwired: 2 out]
      }
      frame "开启阀门" {
      }
    }
    n229 = Empty String/Path?(string/path=w57) -> (empty?=w59:bool)
    n230 = Empty String/Path?(string/path=w65) -> (empty?=w66:bool)
    n231 = case shown="True" w59 {
      tunnel: w58 -> [_ w75]
      tunnel: w57 -> [_ w74]
      tunnel: w56 -> [_ w73]
      frame True {
      }
      frame False {
        n232 = Send Notification(notification=w74, notifier=w75, error in (no error)=w73) -> ()  [unwired: 2 out]
      }
    }
    n233 = case shown="False" w66 {
      tunnel: w72 -> [_ w78]
      tunnel: w65 -> [_ w77]
      tunnel: w60 -> [_ w76]
      frame True {
      }
      frame False {
        n234 = Send Notification(notification=w77, notifier=w78, error in (no error)=w76) -> ()  [unwired: 2 out]
      }
    }
    n235 = global read "退出所有.vi" "退出所有"() -> (w69:bool)
    n236 = local read "Boolean"() -> (w68:bool)
    n237 = Or(x=w69, y=w68) -> (x .or. y?=w67:bool)
  }
